vi "Get Error.vi"(11 "Dev Panel in":refnum<class "Dev Panel.lvclass">) -> (2 "Error":errorcluster)   [LabVIEW 2021, in "Dev Panel.lvclass"]
uses:
  Dev Panel.lvclass
  Dev Panel.lvclass/Dev Panel.ctl
  Actor/Event Actor/Event Actor.lvclass
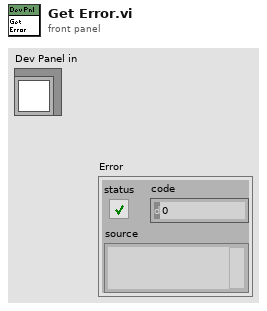
[diagram p1: front panel]
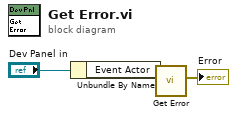
[diagram p0: block diagram]
diagram:
  n1 = Unbundle By Name("Dev Panel in") -> ("Event Actor"=w1:refnum<class "Event Actor.lvclass">)
  n2 = call-dynamic "Get Error.vi"("Actor in"=w1) -> ("Error"=→"Error":errorcluster)  [unwired: 10 in]
